vi "GOOP_CreateGoop4Probe.vi"(7 "LVProbeTemp":path, 8 "error in (no error)":errorcluster, 10 "ClassNames":string[](array[string]), 11 "MD5":string) -> (0 "error out":errorcluster, 3 "CacheVI-NameOut":path)   [LabVIEW 2014]
doc: "Create Prove VI if needed, should NOT be reentrant"
uses:
  <vilib>/Utility/miscctls.llb/LVPositionTypeDef.ctl
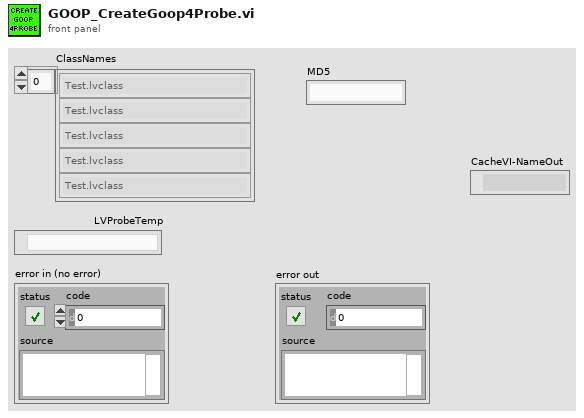
[diagram p1: front panel]
types:
  T1 = enum16{"Share clones between instances", "Preallocate clone for each instance"}
  T2 = typedef "LVPositionTypeDef.ctl" = cluster{"Left":i32, "Top":i32}
  T3 = enum32{"not a typedef", "typedef", "strict typedef", "class private data"}
  T4 = typedef "LVRectTypeDef.ctl" = cluster{"Left":i16, "Top":i16, "Right":i16, "Bottom":i16}
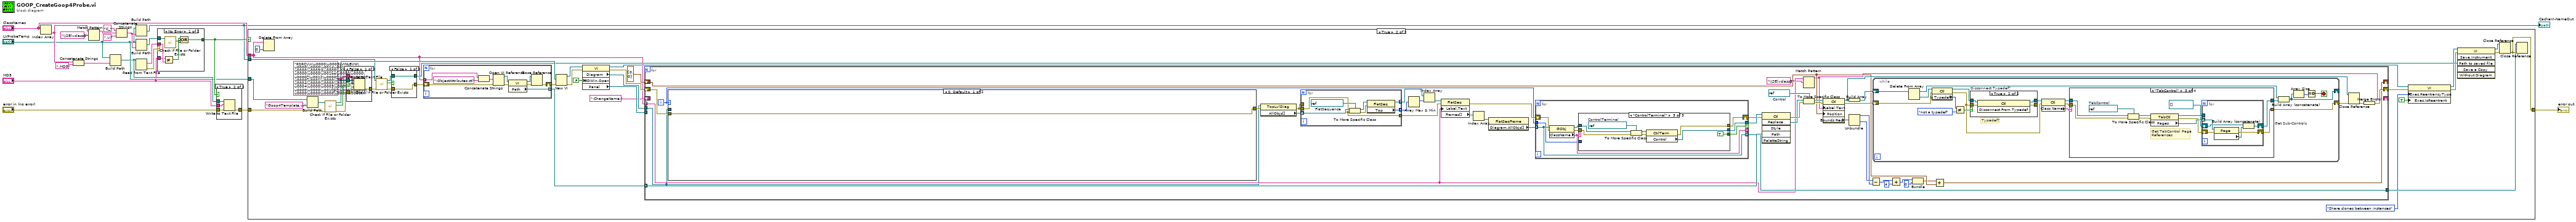
[diagram p0: block diagram]
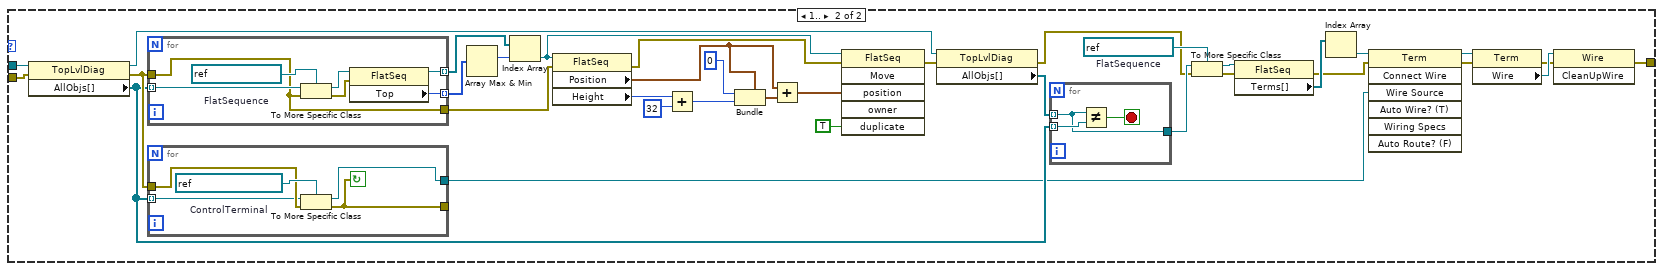
[diagram p3: hidden frame]
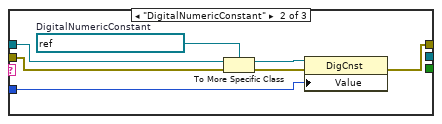
[diagram p5: hidden frame]
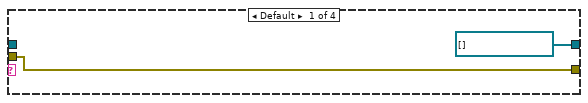
[diagram p7: hidden frame]
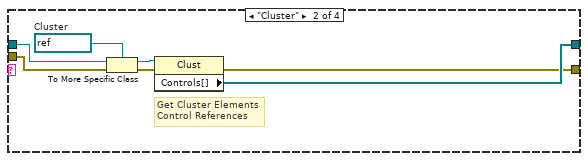
[diagram p8: hidden frame]
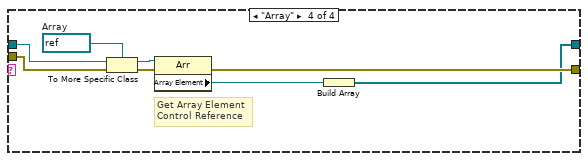
[diagram p9: hidden frame]
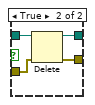
[diagram p10: hidden frame]
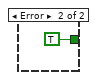
[diagram p13: hidden frame]
diagram:
  n1 = Index Array(array="ClassNames") -> (element=w15:string)  [unwired: 1 in]
  n2 = Concatenate Strings(w15, ".MD5" ("string")) -> (w19:string)
  n3 = Match Pattern(string=w15, regular expression="\\2Elvclass$") -> (before substring=w12:string)  [unwired: 1 in, 3 out]
  n4 = Build Path(base path="LVProbeTemp", name or relative path=w19) -> (appended path=w11:path)
  n5 = Concatenate Strings("C_" ("string"), w12, ".vi" ("string")) -> (w3:string)
  n6 = Build Path(base path="LVProbeTemp", name or relative path=w3) -> (appended path=w2:path)
  "CacheVI-NameOut" <- w2
  n7 = Build Path(base path="LVProbeTemp", name or relative path=w3) -> (appended path=w10:path)
  n8 = Read from Text File(file (use dialog)=w11) -> (text=w17:string, error out=w18:errorcluster)  [unwired: 3 in, 2 out]
  n9 = case shown="No Error" w18 {
    tunnel: [w22 TRUE] -> w7
    tunnel: w17 -> [w26 _]
    tunnel: "MD5" -> [w25 _]
    tunnel: w10 -> [w23 _]
    frame No Error {
      n10 = Not Equal?(x=w25, y=w26) -> (x != y?=w24:bool)
      n11 = call <vilib>:"Check if File or Folder Exists.vi"("path"=w23) -> ("file or folder exists?"=w21:bool)  [unwired: 8 in, 2 out]
      n12 = Compound Arithmetic op=OR(w24, invert w21) -> (w22:bool)
    }
    frame Error {
    }
  }
  n13 = case shown="True" w7 {
    tunnel: w11 -> [_ w32]
    tunnel: "MD5" -> [_ w31]
    tunnel: "error in (no error)" -> [w28 w30]
    tunnel: [w28 w29] -> w5
    frame False {
    }
    frame True {
      n14 = Write to Text File(file (use dialog)=w32, text=w31, error in=w30) -> (error out=w29:errorcluster)  [unwired: 1 in, 2 out]
    }
  }
  n15 = case shown="True" w7 {
    tunnel: "ClassNames" -> [_ w38]
    tunnel: w5 -> [w33 w37]
    tunnel: [w33 w36] -> w4
    tunnel: w2 -> [_ w35]
    tunnel: "LVProbeTemp" -> [_ w34]
    frame False {
    }
    frame True {
      n16 = Delete From Array(array=w38, index=0) -> ()  [unwired: 1 in, 2 out]
      n17 = Build Path(base path=w34, name or relative path="Goop4Template.vi") -> (appended path=w69:path)
      n18 = call <vilib>:"Check if File or Folder Exists.vi"("error in (no error)"=w37, "path"=w69) -> ("error out"=w67:errorcluster, "file or folder exists?"=w45:bool, "dup path"=w66:path)  [unwired: 7 in]
      n19 = case shown="False" w45 {
        tunnel: w66 -> [w274 _]
        tunnel: "RSRC\r\n\u0000\u0003LVINLBVW\u0000\u0000\u001c\u0018\u0000\u0000\u0003\t\u0000\u0000\u0000 \u0000\u0000\u001bø\u0000\u0000\u0000\u0012\u0000\u0004\u0000\u0000\u0001\u0000\u0000\u0000\u0004\u0000\u0000\u0000\u0000\u0004\u0000\u0003\u0000<\u0000\u0000\u0000\u001f@\u0002\u0010\u0000\u0000\u0000\u0001\u0000\u0001\u0000\u0002ÿÿÿÿ\u0000\u0000\u0000\u0000\u0000\u0000\u0000\u0000\u0000\u0000\u0000\u0000VK`ËÿçFÜEÂ\u0013\u001dëÊ\u0000\u0000\u0000\f\u0000\u0000\u0000\u0010\u0000\u0000\u0000\u0000Ï_\u0016t4³pNAL\u0012°aÔ\u001dÙ\u0000²\u0004é\tìøB~\u0000\u0000\u0010\u0000\u0000\u0000\u0000\u0000OGñå§ZqF°K\u0011nô\u0016\u0000\u0000\u0000\u0010j\u001dþáñÎi\u001b\u001e1\u0012Yê#\"\u0000\u0000\u0000\f\u0012\u0000$\u0000\u0000\u000412.0\u0000\u0000\u0000\u0000\u0002\u0000\u0001\u0000\u0000\u0000\u0000\u0000 \u0000\u0001LVIN\u0010Goop4Template.vi\u0000\u0000\u0000\u0000\u0000\u0000\u0000\u0000\u0003\u0000\u0000\u00000Ô\u001dÙ\u0000²\u0004é\tìøB~å\u001dFú\tÔ\nvV\u000e©øÄÖÂüáÕ¾qÕwJ\u0012Âí^c\u0000\u0000\u0000ÿÿÿÿ\u0000\u0000\u0001\u0000\u0000\u0001\u0000\u0000\u0001\u0000\u0000\u0001\u0000\u0000\u0001\u0000\u0000\u00011\u0011JR1J\\QJPq1\u0011\u0000\u0000\u0001\u0000\u0000\u0001\u0000\u0000\u0001\u0000\u0000\u0001\u0000\u0000\u0001\u0000\u0000\u0001\u0000\u0000\u0001qáJRr\\ÁJRIá\u0000\u0000\u0001\u0000\u0000\u0001\u0000\u0000\u0001\u0000\u0000\u0001\u0000\u0000\u0001\u0000\u0000\u0001\u0000\u0000\u0001ÿÿÿÿ\u0000\u0000\u0002\u0000ÿÿÿÿÿÿÿÿÿÿÿÿÿÿÿÿøøøøøøøÿÿøÿøøøøøÿøøÿøøÿ..." ("text") -> [w273 _]
        tunnel: w67 -> [w272 w275]
        tunnel: [w271 w275] -> w51
        frame False {
          n20 = Write to Text File(file (use dialog)=w274, text=w273, error in=w272) -> (error out=w271:errorcluster)  [unwired: 1 in, 2 out]
        }
        frame True {
        }
      }
      n21 = call <vilib>:"Check if File or Folder Exists.vi"("error in (no error)"=w51, "path"=w35) -> ("error out"=w52:errorcluster, "file or folder exists?"=w65:bool, "dup path"=w64:path)  [unwired: 7 in]
      n22 = case shown="False" w65 {
        tunnel: w64 -> [w266 w270]
        tunnel: [w266 w269] -> w60
        tunnel: w52 -> [w265 w268]
        tunnel: [w265 w267] -> w50
        frame False {
        }
        frame True {
          n23 = Delete(path (use dialog)=w270, error in=w268) -> (deleted path=w269:path, error out=w267:errorcluster)  [unwired: 3 in, 1 out]
        }
      }
      n24 = for {
        tunnel: [w73] -> w57 mode=indexing
        tunnel: w38 -> [w71] mode=indexing
        shift-right: [w74] -> w58
        shift-left: w50 -> [w72]
        n25 = Concatenate Strings(w71, ":ObjectAttributes.ctl" ("string")) -> (w79:string)
        n26 = Open VI Reference(vi path=w79, error in (no error)=w72) -> (vi reference=w78:refnum<vi>, error out=w77:errorcluster)  [unwired: 4 in]
        n27 = property class="VI"(reference=w78, error in=w77) -> (reference out=w75:refnum<vi>, error out=w76:errorcluster, "Path"=w73:path)
        n28 = Close Reference(reference=w75, error in (no error)=w76) -> (error out=w74:errorcluster)
      }
      n29 = New VI(8:w58, 10:w66) -> (0:w63:errorcluster, 3:w48:refnum<vi>)  [unwired: 5 in]
      n30 = property class="VI"(reference=w48, error in=w63, "BDWin.Open"=FALSE ("Block Diagram Window:Open")) -> (reference out=w43:refnum<vi>, error out=w55:errorcluster, "Diagram"=w62:refnum<vi>, "Panel"=w59:refnum<vi>)
      n31 = for {
        tunnel: w62 -> [w101]
        tunnel: w59 -> [_]
        tunnel: w57 -> [w123] mode=indexing
        tunnel: [w108] -> w54
        tunnel: w38 -> [w102] mode=indexing
        shift-right: [w122] -> w56
        shift-left: w55 -> [w105]
        shift-right: [w91] -> _
        shift-left: T2 {"Left"=0, "Top"=0} ("Position") -> [w94]
        shift-right: [w90] -> _
        shift-left: ":ChangeName:" ("y") -> [_]
        i -> [w106]
        w121 = refnum<vi> refnum  # Control
        n32 = case shown="0, Default" w106 {
          tunnel: w105 -> [w131 w164]
          tunnel: [w131 w136] -> w104
          tunnel: w101 -> [_ w166]
          frame 0, Default {
          }
          frame 1.. {
            w151 = refnum<vi> refnum  # FlatSequence
            n33 = property class="TopLvlDiag"(reference=w166, error in=w164) -> (reference out=w153:refnum<vi>, error out=w148:errorcluster, "AllObjs[]"=w147:refnum<vi>[])
            n34 = for {
              tunnel: w147 -> [w180] mode=indexing
              tunnel: w148 -> [w177]
              tunnel: [w177] -> w163
              tunnel: [w176] -> w135 mode=indexing
              tunnel: [w175] -> w134 mode=indexing
              w181 = refnum<vi> refnum  # FlatSequence
              n35 = To More Specific Class(target class=w181, reference=w180, error in=w177) -> (specific class reference=w179:refnum<vi>, error out=w178:errorcluster)
              n36 = property class="FlatSeq"(reference=w179, error in=w178) -> (reference out=w175:refnum<vi>, "Top"=w176:i32)  [unwired: 1 out]
            }
            n37 = for {
              tunnel: [w171] -> w142
              tunnel: w147 -> [w168] mode=indexing
              tunnel: w148 -> [w169]
              tunnel: [w167] -> _
              stop <- w167 continue-if-true
              w170 = refnum<vi> refnum  # ControlTerminal
              n38 = To More Specific Class(target class=w170, reference=w168, error in=w169) -> (specific class reference=w171:refnum<vi>, error out=w167:errorcluster)
            }
            n39 = Array Max & Min(array=w135) -> (max index (indices)=w133:i32)  [unwired: 3 out]
            n40 = Index Array(array=w134, index=w133) -> (element=w132:refnum<vi>)
            n41 = property class="FlatSeq"(reference=w132, error in=w163) -> (error out=w155:errorcluster, "Position"=w160:T2, "Height"=w158:u32)  [unwired: 1 out]
            n42 = Add(x=w158, y=32 ("Left")) -> (x+y=w156:u32)
            n43 = Bundle(cluster=w160, "Left"=0, "Top"=w156) -> (w161:T2)
            n44 = Add(x=w160, y=w161) -> (x+y=w162:T2)
            n45 = invoke class="FlatSeq" method="Move"(reference=w132, error in=w155, "position"=w162, "duplicate"=TRUE ("Duplicate? (F)")) -> (error out=w154:errorcluster)  [unwired: 2 in, 5 out]
            n46 = property class="TopLvlDiag"(reference=w153, error in=w154) -> (error out=w149:errorcluster, "AllObjs[]"=w152:refnum<vi>[])  [unwired: 1 out]
            n47 = for {
              tunnel: w152 -> [w172] mode=indexing
              tunnel: w147 -> [w174] mode=indexing
              tunnel: [w172] -> w150
              stop <- w173 stop-if-true
              n48 = Not Equal?(x=w172, y=w174) -> (x != y?=w173:bool)
            }
            n49 = To More Specific Class(target class=w151, reference=w150, error in=w149) -> (specific class reference=w146:refnum<vi>, error out=w145:errorcluster)
            n50 = property class="FlatSeq"(reference=w146, error in=w145) -> (error out=w141:errorcluster, "Terms[]"=w144:refnum<vi>[])  [unwired: 1 out]
            n51 = Index Array(array=w144) -> (element=w143:refnum<vi>)  [unwired: 1 in]
            n52 = invoke class="Term" method="Connect Wire"(reference=w143, error in=w141, "Wire Source"=w142) -> (reference out=w140:refnum<vi>, error out=w139:errorcluster)  [unwired: 4 in, 5 out]
            n53 = property class="Term"(reference=w140, error in=w139) -> (error out=w137:errorcluster, "Wire"=w138:refnum<vi>)  [unwired: 1 out]
            n54 = invoke class="Wire" method="CleanUpWire"(reference=w138, error in=w137) -> (error out=w136:errorcluster)  [unwired: 1 in, 2 out]
          }
        }
        n55 = property class="TopLvlDiag"(reference=w101, error in=w104) -> (error out=w83:errorcluster, "AllObjs[]"=w86:refnum<vi>[])  [unwired: 1 out]
        n56 = for {
          tunnel: w86 -> [w129] mode=indexing
          tunnel: w83 -> [w126]
          tunnel: [w126] -> w85
          tunnel: [w125] -> w89 mode=indexing
          tunnel: [w124] -> w88 mode=indexing
          tunnel: w83 -> [_]
          w130 = refnum<vi> refnum  # FlatSequence
          n57 = To More Specific Class(target class=w130, reference=w129, error in=w126) -> (specific class reference=w128:refnum<vi>, error out=w127:errorcluster)
          n58 = property class="FlatSeq"(reference=w128, error in=w127) -> (reference out=w124:refnum<vi>, "Top"=w125:i32)  [unwired: 1 out]
        }
        n59 = Array Max & Min(array=w89) -> (max index (indices)=w87:i32)  [unwired: 3 out]
        n60 = Index Array(array=w88, index=w87) -> (element=w84:refnum<vi>)
        n61 = property class="FlatSeq"(reference=w84, error in=w85, "Label.Text"=w102) -> (error out=w107:errorcluster, "Frames[]"=w111:refnum<vi>[])  [unwired: 1 out]
        n62 = Index Array(array=w111) -> (element=w110:refnum<vi>)  [unwired: 1 in]
        n63 = property class="FlatSeqFrame"(reference=w110) -> ("Diagram.AllObjs[]"=w109:refnum<vi>[])  [unwired: 1 in, 2 out]
        n64 = for {
          tunnel: w109 -> [w188] mode=indexing
          tunnel: [w190] -> _ mode=indexing
          tunnel: [w188] -> w108 mode=indexing
          tunnel: w106 -> [w187]
          shift-right: [w184] -> w81
          shift-left: w107 -> [w186]
          tunnel: [w183] -> w82 if=w182
          n65 = property class="GObj"(reference=w188, error in=w186) -> (reference out=w189:refnum<vi>, error out=w185:errorcluster, "ClassName"=w190:string)
          n66 = case shown="\"ControlTerminal\"" w190 {
            tunnel: w189 -> [_ w198 w206]
            tunnel: w187 -> [_ w197 _]
            tunnel: w185 -> [w191 w194 w203]
            tunnel: [w191 w192 w201] -> w184
            tunnel: [_ _ w200] -> w183
            tunnel: [_ _ TRUE] -> w182
            frame Default {
            }
            frame "DigitalNumericConstant" {
              w196 = refnum<vi> refnum  # DigitalNumericConstant
              n67 = To More Specific Class(target class=w196, reference=w198, error in=w194) -> (specific class reference=w195:refnum<vi>, error out=w193:errorcluster)
              n68 = property class="DigCnst"(reference=w195, error in=w193, "Value"=w197) -> (error out=w192:errorcluster)  [unwired: 1 out]
            }
            frame "ControlTerminal" {
              w205 = refnum<vi> refnum  # ControlTerminal
              n69 = To More Specific Class(target class=w205, reference=w206, error in=w203) -> (specific class reference=w204:refnum<vi>, error out=w202:errorcluster)
              n70 = property class="CtrlTerm"(reference=w204, error in=w202) -> (error out=w201:errorcluster, "Control"=w200:refnum<vi>)  [unwired: 1 out]
            }
          }
        }
        n71 = invoke class="Ctl" method="Replace"(reference=w82, error in=w81, "Path"=w123) -> (error out=w117:errorcluster, "Replace"=w118:refnum<vi>)  [unwired: 3 in, 4 out]
        n72 = Match Pattern(string=w102, regular expression="\\2Elvclass$") -> (before substring=w90:string)  [unwired: 1 in, 3 out]
        n73 = To More Specific Class(target class=w121, reference=w118, error in=w117) -> (specific class reference=w115:refnum<vi>, error out=w113:errorcluster)
        n74 = property class="Ctl"(reference=w115, error in=w113, "Label.Text"=w90, "Position"=w94) -> (reference out=w114:refnum<vi>, error out=w112:errorcluster, "Bounds Rect"=w100:T4)
        n75 = Build Array(w114) -> (w120:refnum<vi>[])
        n76 = Unbundle(w100) -> ("Left"=w98:i16, "Right"=w99:i16)  [unwired: 2 out]
        n77 = Subtract(x=w99, y=w98) -> (x-y=w97:i16)
        n78 = while {
          shift-right: [w216] -> _
          shift-left: w120 -> [w219]
          shift-right: [w220] -> w119
          shift-left: w112 -> [w211]
          stop <- w214 stop-if-true
          # "Typedef?"
          n79 = Delete From Array(array=w219) -> (deleted portion=w213:refnum<vi>, array with subset deleted=w218:refnum<vi>[])  [unwired: 2 in]
          n80 = property class="Ctl"(reference=w213, error in=w211) -> (reference out=w212:refnum<vi>, error out=w207:errorcluster, "Is Typedef?"=w210:T3)
          n81 = Not Equal?(x=w210, y=T3."not a typedef") -> (x != y?=w209:bool)
          n82 = case "Disconnect Typedef?" shown="True" w209 {
            tunnel: [w225 w230] -> w217
            tunnel: [w226 w229] -> _
            tunnel: w212 -> [w225 w228]
            tunnel: w207 -> [w226 w227]
            frame False {
            }
            frame True {
              n83 = invoke class="Ctl" method="Disconnect From Typedef"(reference=w228, error in=w227) -> (reference out=w230:refnum<vi>, error out=w229:errorcluster)  [unwired: 1 in, 1 out]
            }
          }
          n84 = property class="Ctl"(reference=w217, error in=w207) -> (reference out=w223:refnum<vi>, error out=w222:errorcluster, "Class Name"=w224:string)
          n85 = case "Get Sub-Controls" shown="\"TabControl\"" w224 {
            tunnel: w223 -> [_ w239 w250 w264]
            tunnel: w222 -> [w232 w236 w247 w261]
            tunnel: [refnum<vi>[] [] ("Controls[]") w234 w241 w257] -> w221
            tunnel: [w232 w233 w240 w259] -> w220
            frame Default {
            }
            frame "Cluster" {
              w237 = refnum<vi> refnum  # Cluster
              # "Get Cluster Elements Control References"
              n86 = To More Specific Class(target class=w237, reference=w239, error in=w236) -> (specific class reference=w238:refnum<vi>, error out=w235:errorcluster)
              n87 = property class="Clust"(reference=w238, error in=w235) -> (error out=w233:errorcluster, "Controls[]"=w234:refnum<vi>[])  [unwired: 1 out]
            }
            frame "TabControl" {
              w248 = refnum<vi> refnum  # TabControl
              # "Get TabControl Page References"
              n88 = To More Specific Class(target class=w248, reference=w250, error in=w247) -> (specific class reference=w249:refnum<vi>, error out=w246:errorcluster)
              n89 = property class="TabCtl"(reference=w249, error in=w246) -> (reference out=w244:refnum<vi>, error out=w245:errorcluster, "Pages"=w243:refnum<vi>[])
              n90 = for {
                tunnel: w244 -> [_]
                tunnel: w243 -> [w255] mode=indexing
                shift-right: [w252] -> w241
                shift-left: refnum<vi>[] [] -> [w253]
                shift-right: [w251] -> w240
                shift-left: w245 -> [w256]
                n91 = property class="Page"(reference=w255, error in=w256) -> (error out=w251:errorcluster, "Controls on Page[]"=w254:refnum<vi>[])  [unwired: 1 out]
                n92 = Build Array (concatenate)(w253, w254) -> (w252:refnum<vi>[])
              }
            }
            frame "Array" {
              w262 = refnum<vi> refnum  # Array
              # "Get Array Element Control Reference"
              n93 = To More Specific Class(target class=w262, reference=w264, error in=w261) -> (specific class reference=w263:refnum<vi>, error out=w260:errorcluster)
              n94 = property class="Arr"(reference=w263, error in=w260) -> (error out=w259:errorcluster, "Array Element"=w258:refnum<vi>)  [unwired: 1 out]
              n95 = Build Array(w258) -> (w257:refnum<vi>[])
            }
          }
          n96 = Build Array (concatenate)(w218, w221) -> (w216:refnum<vi>[])
          n97 = Array Size(array=w216) -> (size(s)=w215:i32)
          n98 = Equal To 0?(x=w215) -> (x = 0?=w214:bool)
        }
        n99 = Add(x=w97, y=i16 4) -> (x+y=w95:i16)
        n100 = Bundle(w95, "Left"=0) -> (w93:cluster{i16, "Left":i32})  [unwired: 1 in]
        n101 = Add(x=w93, y=w94) -> (x+y=w91:T2)
        n102 = Close Reference(reference=w114, error in (no error)=w119) -> (error out=w116:errorcluster)
        n103 = Merge Errors(w116) -> (w122:errorcluster)
      }
      n104 = property class="VI"(reference=w43, error in=w56, "Exec.ReentrancyType"=T1."Share clones between instances" ("Execution:Reentrancy Type"), "Exec.IsReentrant"=TRUE ("Execution:Is Reentrant")) -> (reference out=w42:refnum<vi>, error out=w44:errorcluster)
      n105 = invoke class="VI" method="Save.Instrument"(reference=w42, error in=w44, "Path to saved file"=w60) -> (reference out=w40:refnum<vi>, error out=w49:errorcluster)  [unwired: 3 in, 4 out]
      n106 = Close Reference(reference=w40, error in (no error)=w49) -> (error out=w36:errorcluster)
      n107 = Close Reference(reference=w54, error in (no error)=w36) -> ()  [unwired: 1 out]
    }
  }
  "error out" <- w4
